vi "Asynchronous - Detect Change in Array.vi"(8 "Error (in)":errorcluster, 10 "Data (in)":dbl[](array[numeric])) -> (0 "Error (out)":errorcluster, 1 "Indexes":i32[](array[numeric]), 2 "Data (out)":dbl[](array[numeric]))   [LabVIEW 2020, in "Ballard Arinc-429 Engine.lvlib"]
uses:
  Ballard Arinc-429 Engine.lvlib
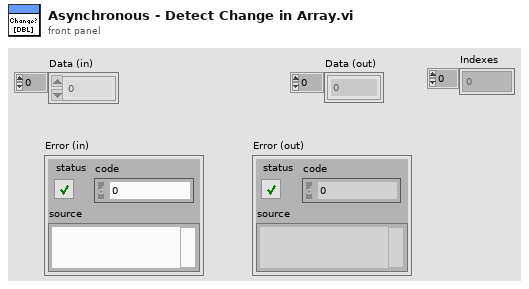
[diagram p1: front panel]
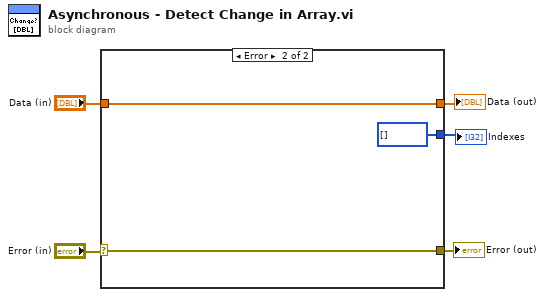
[diagram p0: block diagram]
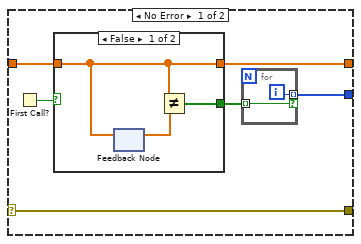
[diagram p2: hidden frame]
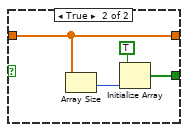
[diagram p3: hidden frame]
diagram:
  n1 = case shown="Error" "Error (in)" {
    selector: "Error (in)" -> [w7 w23]
    tunnel: "Data (in)" -> [w11 w22]
    tunnel: [w9 w22] -> w4
    tunnel: [w7 w23] -> w2
    tunnel: [w6 i32[] []] -> w1
    frame No Error {
      n2 = First Call?() -> (First Call?: T/F=w8:bool)
      n3 = case shown="False" w8 {
        tunnel: w11 -> [w12 w18]
        tunnel: [w13 w15] -> w10
        tunnel: [w12 w18] -> w9
        frame False {
          n4 = feedback #1() -> (w14:dbl[])  [unwired: 1 in]
          n5 = feedback-in #1(w12) -> ()
          n6 = Not Equal?(x=w12, y=w14) -> (x != y?=w13:bool[])
        }
        frame True {
          n7 = Array Size(array=w18) -> (size(s)=w17:i32)
          n8 = Initialize Array(TRUE, w17) -> (w15:bool[])
        }
      }
      n9 = for {
        tunnel: w10 -> [w20] mode=indexing
        tunnel: [w19] -> w6 mode=indexing if=w20
        i -> [w19]
      }
    }
    frame Error {
    }
  }
  "Error (out)" <- w2
  "Data (out)" <- w4
  "Indexes" <- w1
